vi "SetInitialDO.vi"(0 "reference in":refnum<class "Stand.lvclass">, 11 "error in":errorcluster) -> (4 "reference in 2":refnum<class "Stand.lvclass">, 15 "error out":errorcluster)   [LabVIEW 2019, in "Stand.lvclass"]
uses:
  Stand.lvclass
  Stand.lvclass/Stand.ctl
  Sig_DO_Simple_class/Sig_DO_Simple.lvclass/Sig_DO_Simple.ctl
  Proccess_class/Proccess.lvclass/Proccess.ctl
  Sig_AO_class/Sig_AO.lvclass/Sig_AO.ctl
  Logger_class/Logger.lvclass/Logger.ctl
  Sig_DO_Simple_class/private/write_do_to_db.vi
  Sig_AO_class/private/WriteToDb.vi
  Proccess_class/Read TagName.vi
  Proccess_class/Read Logger.vi
  Logger_class/Enqueue Signal.vi
  Sig_DO_Simple_class/Sig_DO_Simple.lvclass
  D:/H4000/src/Proccess_class/Proccess.lvclass
  Sig_AO_class/Sig_AO.lvclass
  Logger_class/WriteEvent.vi
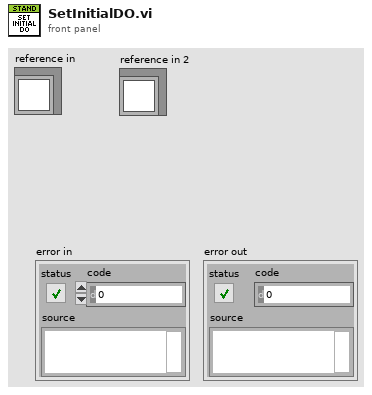
[diagram p1: front panel]
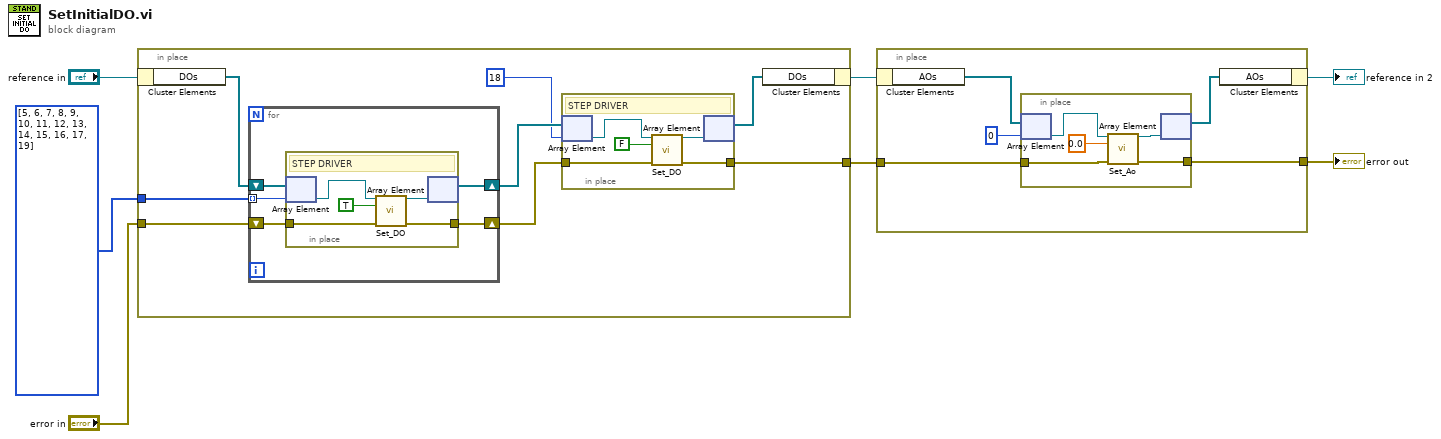
[diagram p0: block diagram]
diagram:
  n1 = in-place {
    in-place-border: "error in" -> [w14]
    in-place-border: [w9] -> w2
    in-place-border: i32[] [5, 6, 7, 8, 9, 10, 11, 12, 13, 14, 15, 16, 17, 19] -> [w13]
    n2 = in-place-cluster #1("reference in") -> ("DOs"=w15:refnum<class "Sig_DO_Simple.lvclass">[])
    n3 = for {
      shift-right: [w22] -> w10
      shift-left: w14 -> [w23]
      shift-right: [w24] -> w12
      shift-left: w15 -> [w25]
      tunnel: w13 -> [w21] mode=indexing
      n4 = in-place {
        in-place-border: w23 -> [w27]
        in-place-border: [w26] -> w22
        # "STEP DRIVER"
        n5 = in-place-array #2(w25, w21) -> (w30:refnum<class "Sig_DO_Simple.lvclass">)
        n6 = call "Set_DO.vi"("reference in"=w30, "DO"=TRUE, "error in (no error)"=w27) -> ("reference out"=w29:refnum<class "Sig_DO_Simple.lvclass">, "error out"=w26:errorcluster)  [unwired: 11 in]
        n7 = in-place-array #2(w29) -> (w24:refnum<class "Sig_DO_Simple.lvclass">[])  [unwired: 1 out]
      }
    }
    n8 = in-place {
      in-place-border: w10 -> [w17]
      in-place-border: [w16] -> w9
      # "STEP DRIVER"
      n9 = in-place-array #3(w12, 18) -> (w20:refnum<class "Sig_DO_Simple.lvclass">)
      n10 = call "Set_DO.vi"("reference in"=w20, "DO"=FALSE, "error in (no error)"=w17) -> ("reference out"=w19:refnum<class "Sig_DO_Simple.lvclass">, "error out"=w16:errorcluster)  [unwired: 11 in]
      n11 = in-place-array #3(w19) -> (w8:refnum<class "Sig_DO_Simple.lvclass">[])  [unwired: 1 out]
    }
    n12 = in-place-cluster #1("DOs"=w8) -> (w4:refnum<class "Stand.lvclass">)
  }
  n13 = in-place {
    in-place-border: w2 -> [w32]
    in-place-border: [w31] -> w1
    n14 = in-place-cluster #4(w4) -> ("AOs"=w35:refnum<class "Sig_AO.lvclass">[])
    n15 = in-place {
      in-place-border: [w37] -> w31
      in-place-border: w32 -> [w36]
      n16 = in-place-array #5(w35, 0) -> (w40:refnum<class "Sig_AO.lvclass">)
      n17 = call "Set_Ao.vi"("reference in"=w40, "AO"=0.0, "error in (no error)"=w36) -> ("reference out"=w38:refnum<class "Sig_AO.lvclass">, "error out"=w37:errorcluster)  [unwired: 11 in]
      n18 = in-place-array #5(w38) -> (w33:refnum<class "Sig_AO.lvclass">[])  [unwired: 1 out]
    }
    n19 = in-place-cluster #4("AOs"=w33) -> (→"reference in 2":refnum<class "Stand.lvclass">)
  }
  "error out" <- w1
